vi "FTW-Endpoint-Multipart-Receive.vi"(0 "FTW Endpoint":refnum<class "FTW-Endpoint.lvclass">, 5 "Timeout":i32 format="%dmsec", 11 "error in":errorcluster) -> (4 "FTW Endpoint out":refnum<class "FTW-Endpoint.lvclass">, 6 "Message Received":string[](array[string]), 8 "Timed out?":bool, 15 "error out":errorcluster)   [LabVIEW 2012, in "FTW-Actor.lvlib" / "FTW-Endpoint.lvclass"]
uses:
  FTW-Endpoint.lvclass
  FTW-Endpoint.lvclass/FTW-Endpoint.ctl
panel:
  # "Inputs"
  # "Outputs"
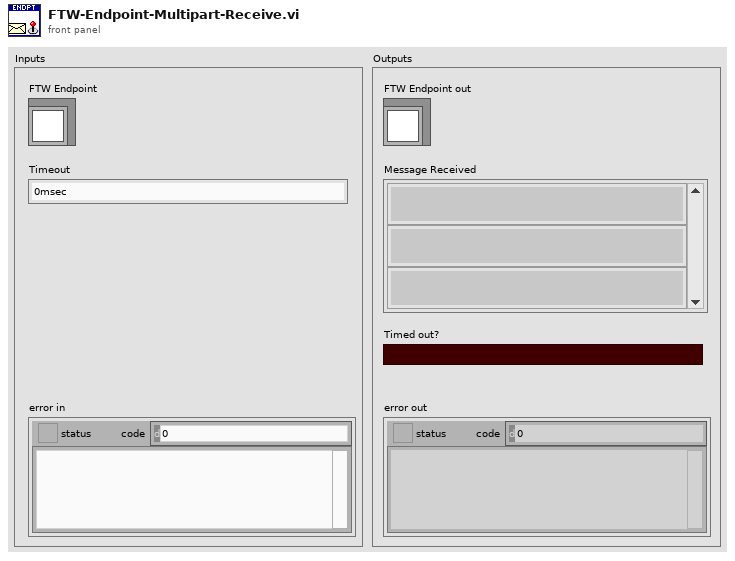
[diagram p1: front panel]
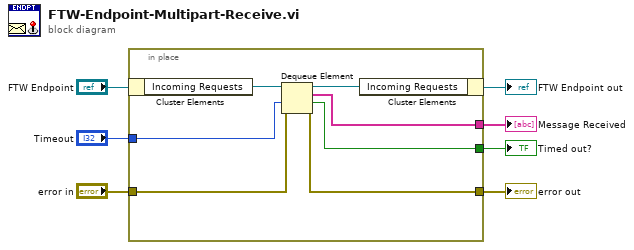
[diagram p0: block diagram]
diagram:
  n1 = in-place {
    in-place-border: [w11] -> w7
    in-place-border: "error in" -> [w12]
    in-place-border: "Timeout" -> [w13]
    in-place-border: [w9] -> w2
    in-place-border: [w8] -> w1
    n2 = in-place-cluster #1("FTW Endpoint") -> ("Incoming Requests"=w14:refnum<queue>)
    n3 = Dequeue Element(queue=w14, timeout in ms (-1)=w13, error in (no error)=w12) -> (queue out=w10:refnum<queue>, element=w9:string[], timed out?=w8:bool, error out=w11:errorcluster)
    n4 = in-place-cluster #1("Incoming Requests"=w10) -> (→"FTW Endpoint out":refnum<class "FTW-Endpoint.lvclass">)
  }
  "error out" <- w7
  "Message Received" <- w2
  "Timed out?" <- w1
